vi "Convert Inches to Revolutions.vi"(10 "Wheel Diameter(in)":dbl=8.0, 11 "Postion(in)":dbl) -> (3 "Revolutions":dbl)   [LabVIEW 2017, in "WCDrive2018.lvlib"]
uses:
  WCDrive2018.lvlib
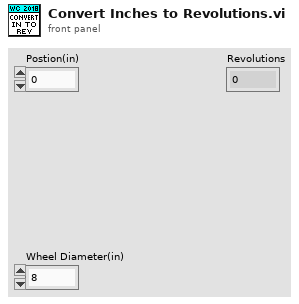
[diagram p1: front panel]
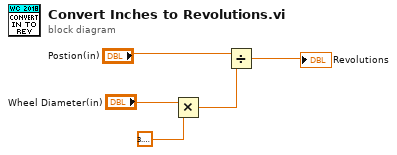
[diagram p0: block diagram]
diagram:
  n1 = Multiply(x="Wheel Diameter(in)", y=3.141592653589793) -> (x*y=w2:dbl)
  n2 = Divide(x="Postion(in)", y=w2) -> (x/y=→"Revolutions":dbl)
